vi "FGV_PCAN_Config.vi"(7 "Write?":bool, 8 "error in":errorcluster caption="错误输入", 9 "FilterMessages":cluster{"Mode: ":T4, "From:":u32, "To:":u32}={"Mode: "=8, "From:"=0, "To:"=0} {"To:" format="%.0x"; "From:" format="%.0x"; "Mode:" items=["PCAN_MODE_STANDARD"=0, "PCAN_MODE_EXTENDED"=2]}, 10 "Initialize":cluster{"Bit rate:":T2, "HwType: ":T3}={"Bit rate:"=9600, "HwType: "=0} {"HwType:" items=["PCAN_TYPE_ISA"=1, "PCAN_TYPE_ISA_SJA"=9, "PCAN_TYPE_ISA_PHYTEC"=4, "PCAN_TYPE_DNG"=2, "PCAN_TYPE_DNG_EPP"=3, "PCAN_TYPE_DNG_SJA"=5, "PCAN_TYPE_DNG_SJA_EPP"=6]; "Bit rate:" items=["PCAN_BAUD_1M"=20, "PCAN_BAUD_800K"=22, "PCAN_BAUD_500K"=28, "PCAN_BAUD_250K"=284, "PCAN_BAUD_125K"=796]}, 11 "Channel":T1 items=["PCAN_USBBUS1"=81, "PCAN_USBBUS2"=82, "PCAN_USBBUS3"=83, "PCAN_USBBUS4"=84]) -> (0 "error out":errorcluster caption="错误输出", 1 "FilterMessages out":cluster{"Mode: ":T4, "From:":u32, "To:":u32}={"Mode: "=8, "From:"=0, "To:"=0} {"To:" format="%.0x"; "From:" format="%.0x"; "Mode:" items=["PCAN_MODE_STANDARD"=0, "PCAN_MODE_EXTENDED"=2]}, 2 "Initialize out":cluster{"Bit rate:":T2, "HwType: ":T3}={"Bit rate:"=9600, "HwType: "=0} {"HwType:" items=["PCAN_TYPE_ISA"=1, "PCAN_TYPE_ISA_SJA"=9, "PCAN_TYPE_ISA_PHYTEC"=4, "PCAN_TYPE_DNG"=2, "PCAN_TYPE_DNG_EPP"=3, "PCAN_TYPE_DNG_SJA"=5, "PCAN_TYPE_DNG_SJA_EPP"=6]; "Bit rate:" items=["PCAN_BAUD_1M"=20, "PCAN_BAUD_800K"=22, "PCAN_BAUD_500K"=28, "PCAN_BAUD_250K"=284, "PCAN_BAUD_125K"=796]}, 3 "Channel out":T1 items=["PCAN_USBBUS1"=81, "PCAN_USBBUS2"=82, "PCAN_USBBUS3"=83, "PCAN_USBBUS4"=84])   [LabVIEW 2020]
uses:
  Window/Control/Bit rate.ctl
  Window/Control/HwType.ctl
  Window/Control/Mode.ctl
  Window/Control/Channel.ctl
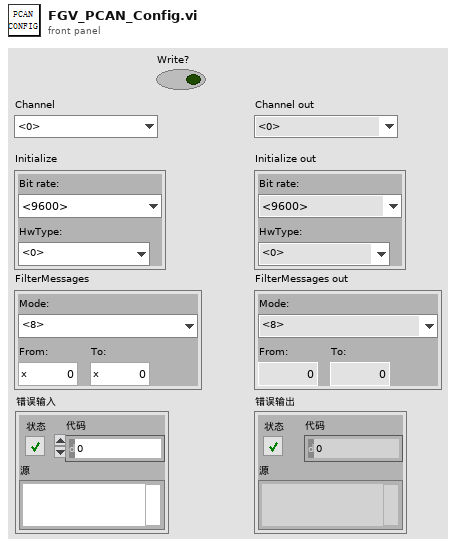
[diagram p1: front panel]
types:
  T1 = typedef "Channel.ctl" = u16
  T2 = typedef "Bit rate.ctl" = u16
  T3 = typedef "HwType.ctl" = u8
  T4 = typedef "Mode.ctl" = u8
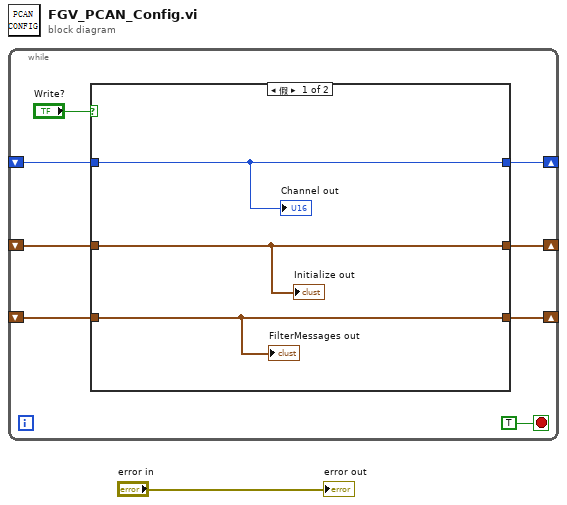
[diagram p0: block diagram]
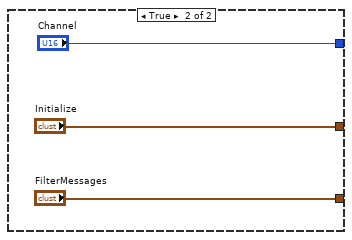
[diagram p2: hidden frame]
diagram:
  n1 = while {
    shift-right: [w8] -> _
    shift-left: _ -> [w6]
    shift-right: [w7] -> _
    shift-left: _ -> [w5]
    shift-right: [w3] -> _
    shift-left: _ -> [w2]
    stop <- TRUE stop-if-true
    n2 = case shown="假" "Write?" {
      tunnel: [w12 "Channel"] -> w8
      tunnel: [w11 "FilterMessages"] -> w7
      tunnel: w6 -> [w12 _]
      tunnel: w5 -> [w11 _]
      tunnel: [w10 "Initialize"] -> w3
      tunnel: w2 -> [w10 _]
      frame False {
        "Channel out" <- w12
        "FilterMessages out" <- w11
        "Initialize out" <- w10
      }
      frame True {
      }
    }
  }
  "error out" <- "error in"
